vi "参数设置页.vi"() -> ()   [LabVIEW 2016, in "斯坦道总磷.lvlib"]
uses:
  <vilib>/Plasmionique/MB Master/MB_Master/MB_Master.lvclass
  <vilib>/ptbypt/NI_PtbyPt.lvlib
panel:
  in  "简易流程周期设置":cluster{"switch button":bool, "设置按钮":bool}
  out "连接状态":bool
  in  "标样核查自动补测":bool caption="通讯连接"
  in  "跨度核查自动补测":bool caption="通讯连接"
  in  "零点核查自动补测":bool caption="通讯连接"
  in  "标样核查标液偏差":dbl caption="标样核查标液偏差："
  in  "跨度核查标液偏差":dbl caption="跨度核查标液偏差："
  in  "零点核查标液偏差":dbl caption="零点核查标液偏差："
  out "低量程上限":dbl caption="低量程上限："
  in  "简易流程路径":path=path "data/流程.xml"
  out "数据刷新时间":string
  in  "通讯连接":bool=TRUE
  out "MB table":enum32{"Serial", "TCP"}(tab)
  in  "请选择串口:":refnum<visa-resource-name>
  in  "IP":string="127.0.0.1"
  in  "PORT":string="1001"
  in  "通信方式选择":enum16{"串口", "TCP"}(ring)
  in  "盐度自动补偿：":bool
  out "盐度补偿值":dbl caption="盐度补偿值："
  in  "刷新":bool
  in  "测量模式":T1(ring)
  in  "参数下拉列表":u16(ring)
  in  "量程下拉列表":enum16{"低量程", "高量程"}(ring)
  in  "测试流程路径":path=path "data/流程.xml"
  in  "标样核查量程模式":T2 caption="标样核查："
  in  "加标回收量程模式":T2 caption="加标回收："
  in  "跨度核查量程模式":T2 caption="跨度核查："
  in  "零点核查量程模式":T2 caption="零点核查："
  in  "水样测试量程模式":T2 caption="水样测试："
  out "稀释度":dbl caption="稀释度："
  out "阈值（高->低）":dbl caption="阈值（高->低）："
  out "阈值（低->高）":dbl caption="阈值（低->高）："
  out "量程下限":dbl caption="量程下限："
  out "高量程上限":dbl caption="高量程上限："
  out "检出限":dbl caption="检出限："
  out "曲线截距":dbl caption="曲线截距：" format="%#.6f"
  out "曲线斜率":dbl caption="曲线斜率：" format="%#.6f"
  out "二次多项式系数":dbl caption="二次多项式系数：" format="%#.6f"
  out "消解时长":dbl caption="消解时长："
  out "消解温度":dbl caption="消解温度："
  out "测量精度":u16 caption="测量精度："
  in  "标样核查标液浓度":dbl caption="标样核查标液浓度："
  in  "跨度核查标液浓度":dbl caption="跨度核查标液浓度："
  in  "零点核查标液浓度":dbl caption="零点核查标液浓度："
  in  "跨度值":dbl caption="跨度值："
  # "日质控设置"
  # "关键参数"
  # "连接设置"
  # "mg/L"
  # "mg/L"
  # "mg/L"
  # "mg/L"
  # "±"
  # "%"
  # "%"
  # "流程设置"
  # "简易流程周期设置"
  # "自动测试量程设置"
  # "设置："
  # "mg/L"
  # "ppt"
  # "mg/L"
  # "mg/L"
  # "mg/L"
  # "mg/L"
  # "mg/L"
  # "min"
  # "℃"
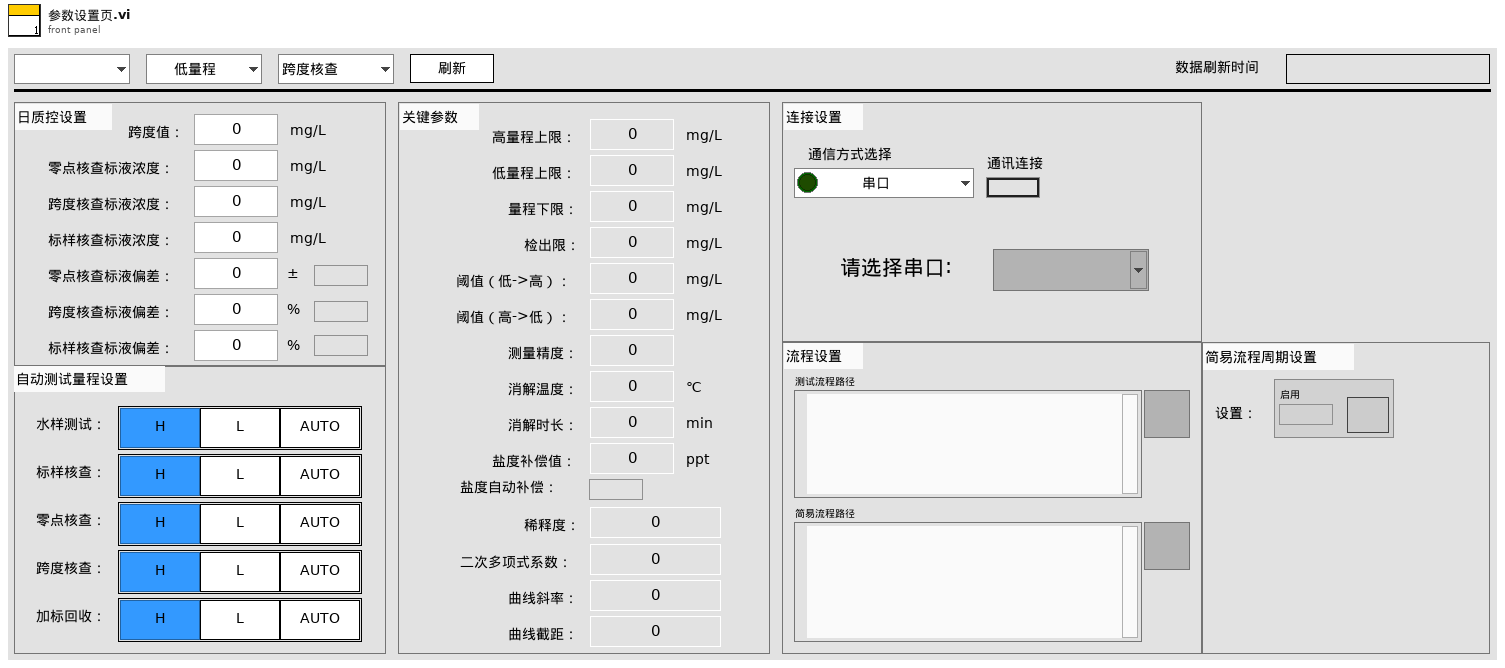
[diagram p1: front panel]
types:
  T1 = enum16{"跨度核查", "水样测量", "零点核查", "标样核查", "加标回收", "快捷测试", "空白校准", "标样校准"}
  T2 = typedef "斯坦道总磷.lvlib/量程模式.ctl" = enum32{"H", "L", "AUTO"}
  T3 = typedef "Cleaning cycle.lvclass/周期项.ctl" = cluster{"时":i32, "分":i32, "频次":string, "id":i32, "参数":string, "simpleflowid":i32, "简易流程名称":string}
  T4 = cluster{"系统时间":timestamp, "工作状态":u16, "测量模式":enum16{"待机", "连续模式", "周期模式", "定点模式", "受控模式", "手动模式"}, "告警代码":u16, "故障代码":u16, "日志代码":u16, "软件版本":u16, "F0":sgl, "F1":sgl, "F2":sgl, "F3":sgl, "T":sgl, "H":sgl, "id":u16, "flowid":u16, "量程":u16, "总磷控温温度1":sgl, "营养盐控温温度2":sgl, "ADC":sgl, "结果值":sgl, "运行时间":u16, "步骤详情":string, "步骤流程":string}
  T5 = typedef "LVStringsAndValuesArrayTypeDef_U16.ctl" = cluster{"String":string, "Value":u16}[]
  T6 = enum8{"Enabled", "Disabled", "Disabled and Grayed Out"}
  T7 = cluster{"测量精度":u16, "检出限":dbl, "上限":dbl, "下限":dbl, "阈值（低->高）":dbl, "阈值（高->低）":dbl, "稀释度":dbl}
  T8 = typedef "操作日志字段定义.ctl" = cluster{"时间":timestamp, "参数":string, "日志信息":string, "流程参数":string}
  T9 = typedef "SingleStepTestV3.lvlib/SingleStepTestV3.lvclass/仪器版本.ctl" = enum16{"V3.1版", "V4版", "V3版", "V4.2版"}
  T10 = typedef "斯坦道总磷.lvlib/V3.1版外设参数.ctl" = cluster{"泵类型":u8, "进样速度":u32, "出样速度":u32, "泵阀量":u8, "阀方向":u8, "光谱仪类型":u8, "光谱采样次数":u8, "氙灯次数":u8, "B":u16, "C":u16, "D":u16, "E":u16, "B_COD":u16, "C_COD":u16, "D_COD":u16, "E_COD":u16, "G":u16, "M":u16, "N":u16, "氨氮注射泵控温下限":sgl, "氨氮注射泵控温上限":sgl, "总氮注射泵控温下限":sgl, "总氮注射泵控温上限":sgl, "消解温度下限":sgl, "消解温度上限":sgl, "加热10s限值":sgl, "KP":sgl, "KI":sgl, "KD":sgl, "高温高压阀开阀温度":sgl, "总氮x公式0":u8, "总氮x公式1":sgl, "总氮x公式2":sgl, "总磷浊度稀释系数":sgl, "总磷浊度补偿权重1":sgl, "总磷浊度补偿权重2":sgl, "盐度系数":sgl, "氨氮补偿系数1":sgl, "氨氮补偿系数2":sgl}
  T11 = typedef "斯坦道总磷.lvlib/V4版外设参数.ctl" = cluster{"泵类型":u8, "注射泵正常速度":u32, "注射泵慢速":u32, "阀型号":u8, "res":u8, "光谱仪类型":u8, "光谱采样次数":u8, "氙灯次数":u8, "B":u16, "C":u16, "D":u16, "E":u16, "B_COD":u16, "C_COD":u16, "D_COD":u16, "E_COD":u16, "G":u16, "M":u16, "N":u16, "降温下限":sgl, "降温上限":sgl, "恒温温度下限":sgl, "恒温温度上限":sgl, "消解温度下限":sgl, "消解温度上限":sgl, "加热10s限值":sgl, "KP":sgl, "KI":sgl, "KD":sgl, "高温高压阀开阀温度":sgl, "总氮x公式0":u8, "总氮x公式1":sgl, "总氮x公式2":sgl, "总磷浊度稀释系数":sgl, "总磷浊度补偿权重1":sgl, "总磷浊度补偿权重2":sgl, "盐度系数":sgl, "氨氮补偿系数1":sgl, "氨氮补偿系数2":sgl, "缺试剂传感器阈值":u16}
  T12 = typedef "斯坦道总磷.lvlib/V4.2版外设参数.ctl" = cluster{"工作模式":u16, "泵类型":u16, "阀型号":u16, "注射泵进样速度":u16, "注射泵出样速度":u16, "注射泵滴定速度":u16, "res":u16, "注射泵慢速":u16, "光谱仪类型":u16, "光谱采样次数":u16, "氙灯次数":u16, "B":u16, "C":u16, "D":u16, "E":u16, "B_COD":u16, "C_COD":u16, "D_COD":u16, "E_COD":u16, "G":u16, "M":u16, "N":u16, "温度校准参数":sgl, "降温温度":sgl, "恒温温度":sgl, "消解温度":sgl, "高温高压阀开阀温度":sgl, "加热超时时间":sgl, "KP":sgl, "KI":sgl, "KD":sgl, "消解PID积分上限":sgl, "恒温PID积分上限":sgl, "PID积分下限":sgl, "缺试剂传感器阈值":u16, "滴定延时":u16, "滴定斜率阈值":sgl, "总氮x公式0":u16, "总氮x公式1":sgl, "总氮x公式2":sgl, "总磷浊度稀释系数":sgl, "总磷浊度补偿权重1":sgl, "总磷浊度补偿权重2":sgl, "盐度系数":sgl, "氨氮补偿系数1":sgl, "氨氮补偿系数2":sgl}
  T13 = typedef "斯坦道总磷.lvlib/V3版外设参数.ctl" = cluster{"泵类型":u8, "进样速度":u32, "出样速度":u32, "泵阀量":u8, "光谱仪类型":u8, "光谱采样次数":u8, "氙灯次数":u8, "B":u16, "C":u16, "D":u16, "E":u16, "B_COD":u16, "C_COD":u16, "D_COD":u16, "E_COD":u16, "G":u16, "M":u16, "N":u16, "氨氮注射泵控温下限":sgl, "氨氮注射泵控温上限":sgl, "总氮注射泵控温下限":sgl, "总氮注射泵控温上限":sgl, "消解温度下限":sgl, "消解温度上限":sgl, "加热10s限值":sgl, "高温高压阀开阀温度":sgl, "总氮x公式0":u8, "总氮x公式1":sgl, "总氮x公式2":sgl, "总磷浊度稀释系数":sgl, "总磷浊度补偿权重1":sgl, "总磷浊度补偿权重2":sgl, "盐度系数":sgl, "氨氮补偿系数1":sgl, "氨氮补偿系数2":sgl}
  T14 = cluster{"水样测试量程模式":T2, "零点核查量程模式":T2, "跨度核查量程模式":T2, "加标回收量程模式":T2, "标样核查量程模式":T2}
  T15 = cluster{"总磷":dbl, "总氮":dbl, "氨氮":dbl, "磷酸盐":dbl, "硝氮":dbl, "亚硝氮":dbl, "硅酸盐":dbl, "硫化物":dbl, "COD":dbl, "氟化物":dbl, "CODMn":dbl}
  T16 = cluster{"总磷跨度值":dbl, "总磷零点标准液浓度":dbl, "总磷跨度标准液浓度":dbl, "总磷标准液标准浓度":dbl, "总氮跨度值":dbl, "总氮零点标准液浓度":dbl, "总氮跨度标准液浓度":dbl, "总氮标准液标准浓度":dbl, "COD跨度值":dbl, "COD零点标准液浓度":dbl, "COD跨度标准液浓度":dbl, "COD标准液标准浓度":dbl, "氨氮跨度值":dbl, "氨氮零点标准液浓度":dbl, "氨氮跨度标准液浓度":dbl, "氨氮标准液标准浓度":dbl, "磷酸盐跨度值":dbl, "磷酸盐零点标准液浓度":dbl, "磷酸盐跨度标准液浓度":dbl, "磷酸盐标准液标准浓度":dbl, "硝氮跨度值":dbl, "硝氮零点标准液浓度":dbl, "硝氮跨度标准液浓度":dbl, "硝氮标准液标准浓度":dbl, "亚硝氮跨度值":dbl, "亚硝氮零点标准液浓度":dbl, "亚硝氮跨度标准液浓度":dbl, "亚硝氮标准液标准浓度":dbl, "硫化物跨度值":dbl, "硫化物零点标准液浓度":dbl, "硫化物跨度标准液浓度":dbl, "硫化物标准液标准浓度":dbl, "硅酸盐跨度值":dbl, "硅酸盐零点标准液浓度":dbl, "硅酸盐跨度标准液浓度":dbl, "硅酸盐标准液标准浓度":dbl, "总磷零点标准液偏差":dbl, "总磷跨度标准液偏差":dbl, "总磷标准液标准偏差":dbl, "总氮零点标准液偏差":dbl, "总氮跨度标准液偏差":dbl, "总氮标准液标准偏差":dbl, "COD零点标准液偏差":dbl, "COD跨度标准液偏差":dbl, "COD标准液标准偏差":dbl, "氨氮零点标准液偏差":dbl, "氨氮跨度标准液偏差":dbl, "氨氮标准液标准偏差":dbl, "磷酸盐零点标准液偏差":dbl, "磷酸盐跨度标准液偏差":dbl, "磷酸盐标准液标准偏差":dbl, "硝氮零点标准液偏差":dbl, "硝氮跨度标准液偏差":dbl, "硝氮标准液标准偏差":dbl, "亚硝氮零点标准液偏差":dbl, "亚硝氮跨度标准液偏差":dbl, "亚硝氮标准液标准偏差":dbl, "硫化物零点标准液偏差":dbl, "硫化物跨度标准液偏差":dbl, "硫化物标准液标准偏差":dbl, "硅酸盐零点标准液偏差":dbl, "硅酸盐跨度标准液偏差":dbl, "硅酸盐标准液标准偏差":dbl, "氟化物跨度值":dbl, "氟化物零点标准液浓度":dbl, "氟化物跨度标准液浓度":dbl, "氟化物标准液标准浓度":dbl, "氟化物零点标准液偏差":dbl, "氟化物跨度标准液偏差":dbl, "氟化物标准液标准偏差":dbl, "CODMn跨度值":dbl, "CODMn零点标准液浓度":dbl, "CODMn跨度标准液浓度":dbl, "CODMn标准液标准浓度":dbl, "CODMn零点标准液偏差":dbl, "CODMn跨度标准液偏差":dbl, "CODMn标准液标准偏差":dbl}
  T17 = cluster{"水样测试量程模式":enum16{"H", "L", "AUTO"}, "空白核查量程模式":enum16{"H", "L", "AUTO"}, "跨度核查量程模式":enum16{"H", "L", "AUTO"}, "加标回收量程模式":enum16{"H", "L", "AUTO"}, "标样核查量程模式":enum16{"H", "L", "AUTO"}}
  T18 = cluster{"水样测试量程模式":u16, "空白核查量程模式":u16, "跨度核查量程模式":u16, "加标回收量程模式":u16, "标样核查量程模式":u16}
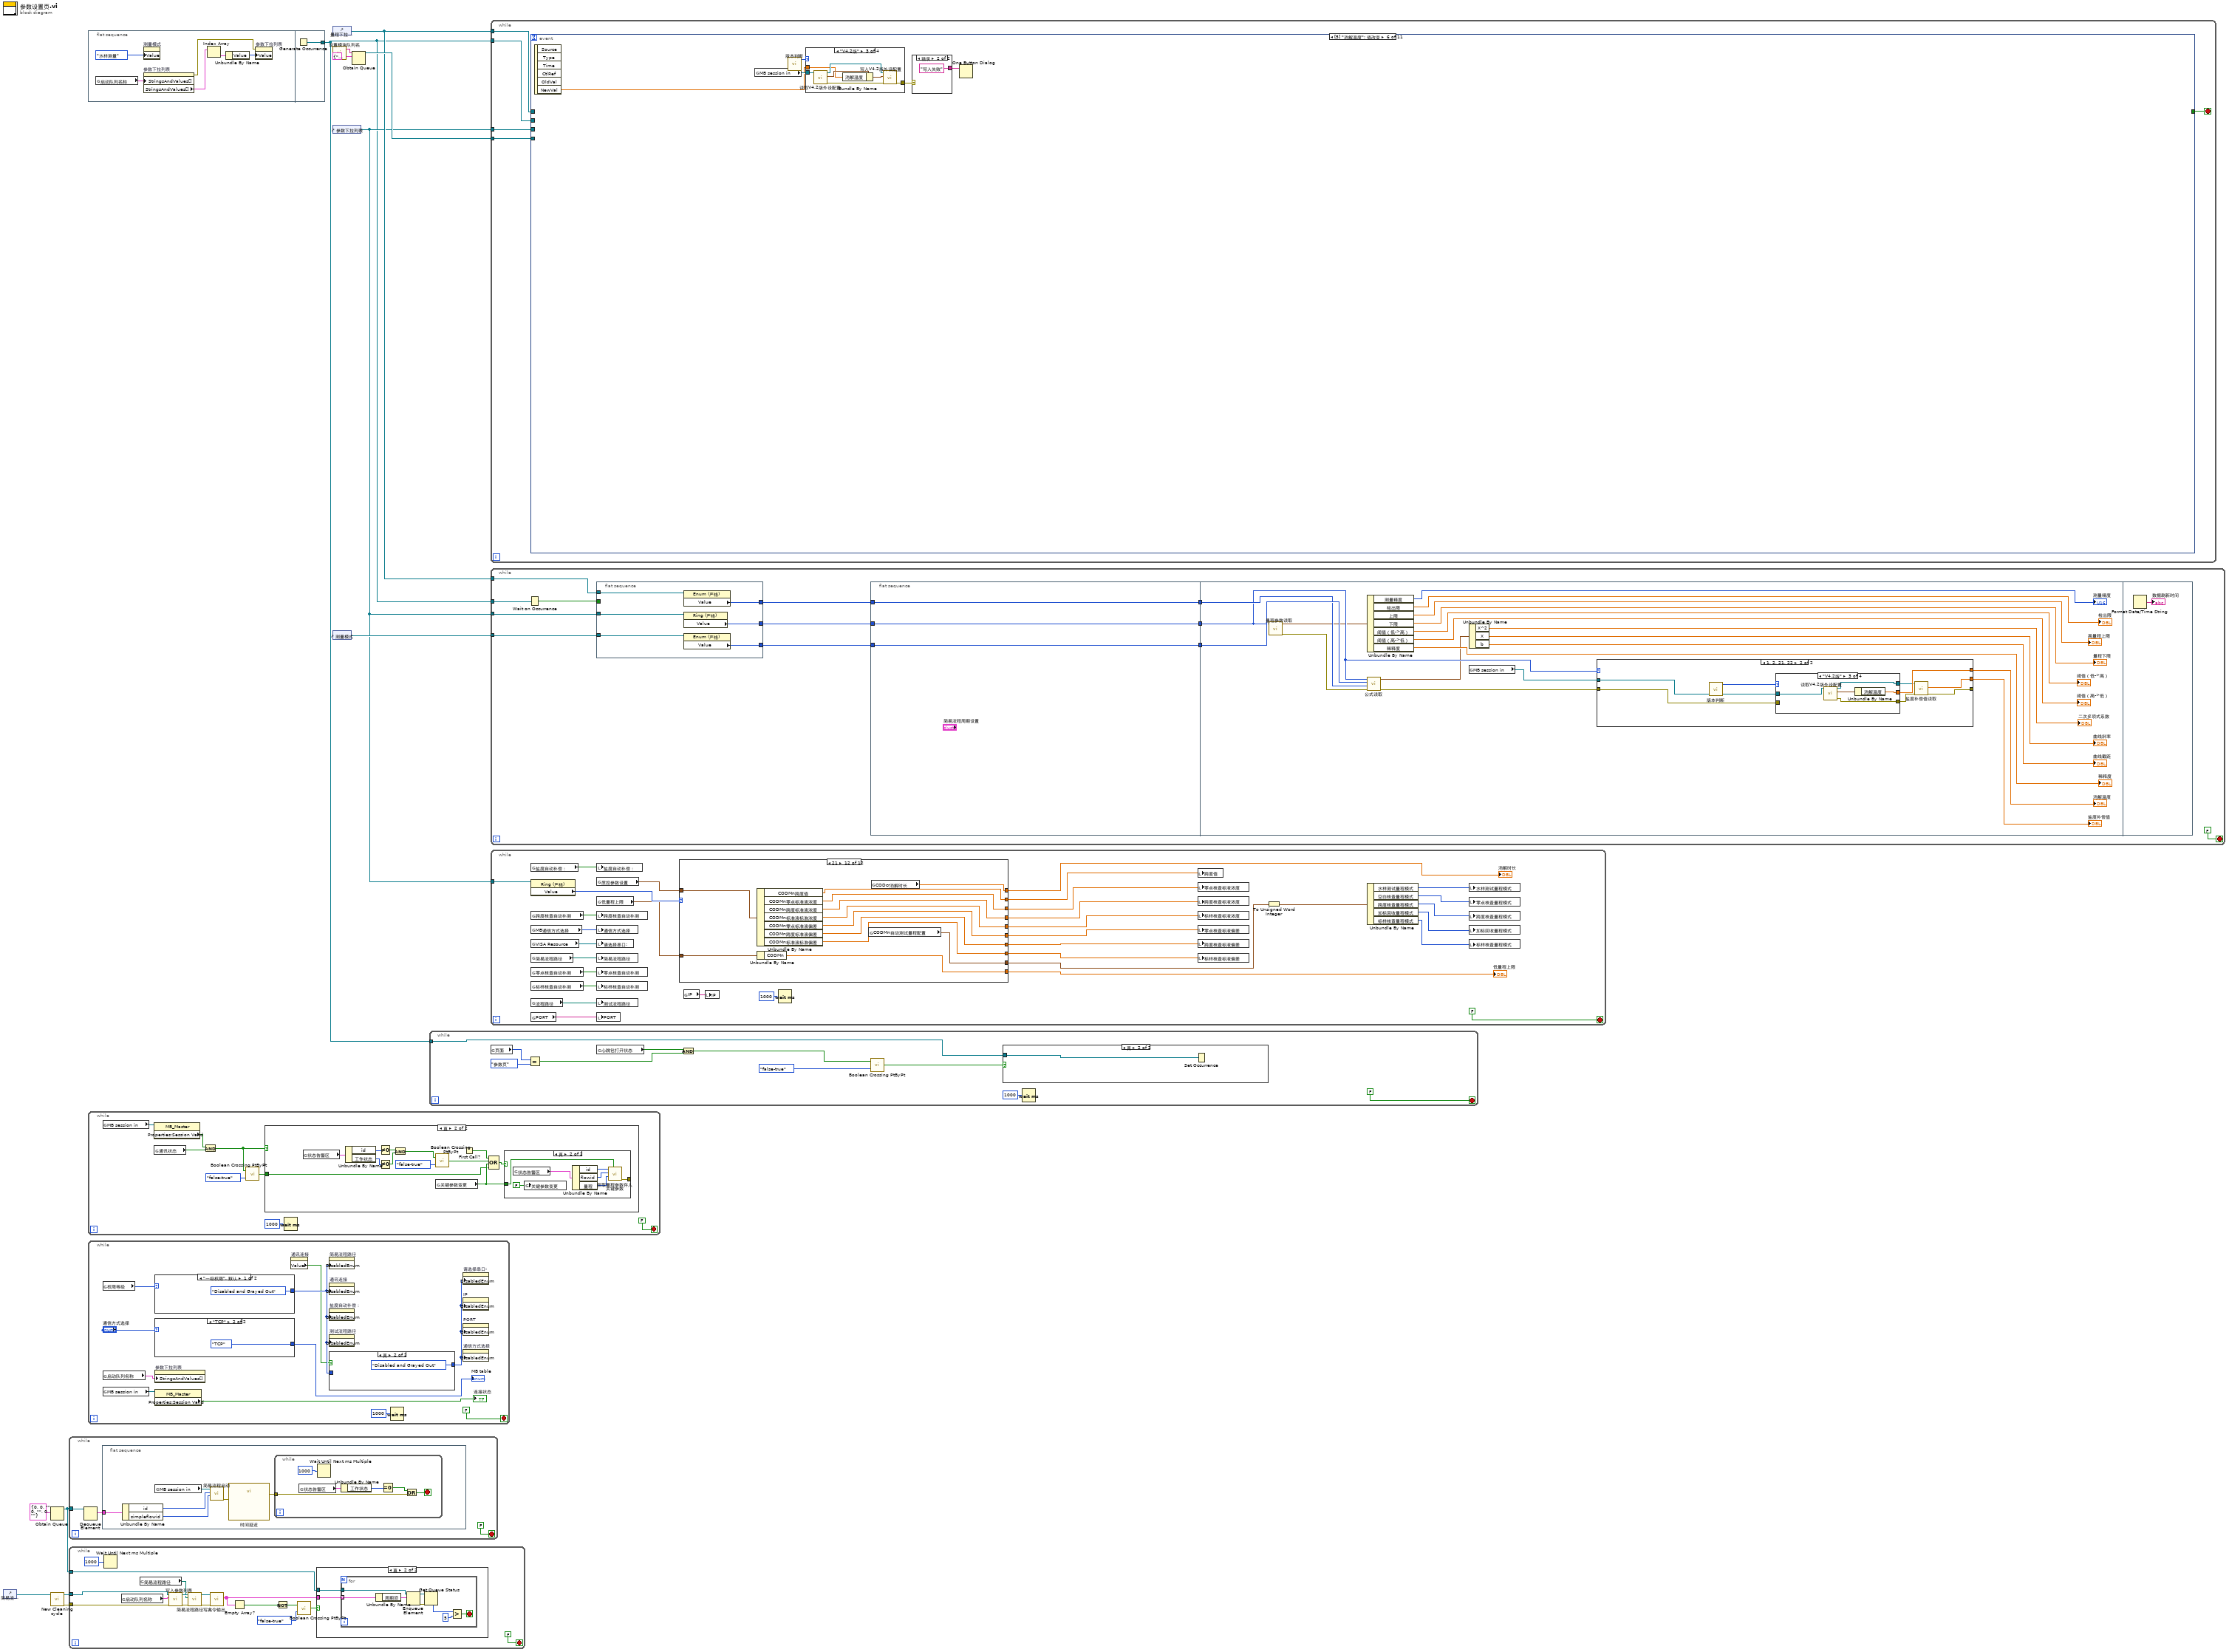
[diagram p0: block diagram]
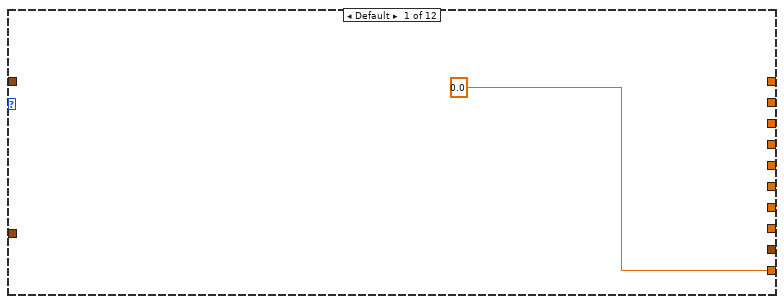
[diagram p6: hidden frame]
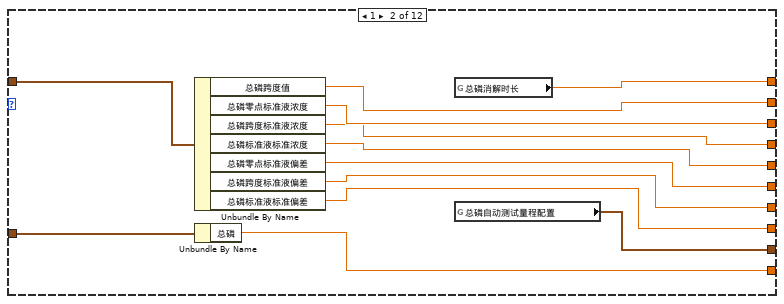
[diagram p7: hidden frame]
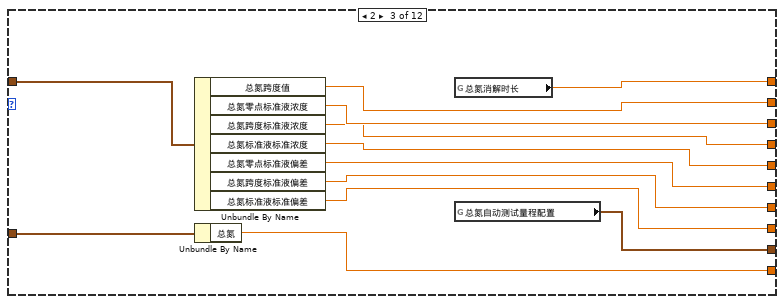
[diagram p8: hidden frame]
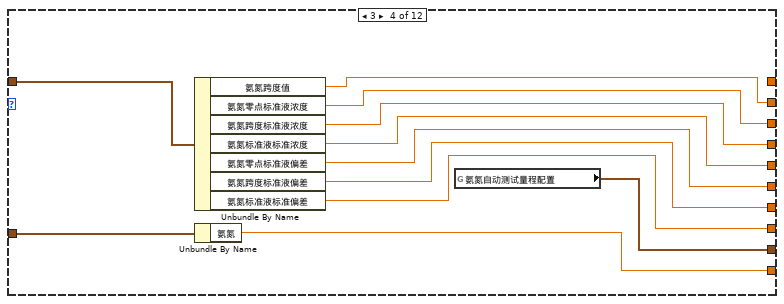
[diagram p9: hidden frame]
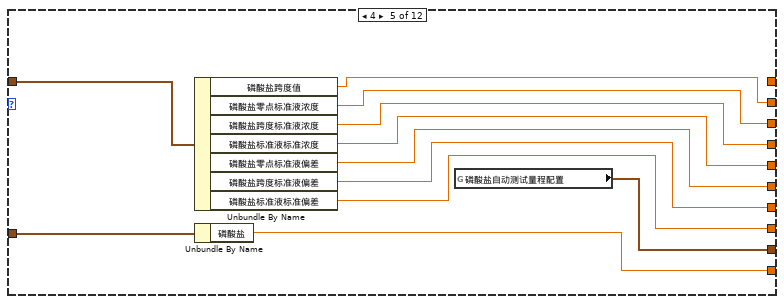
[diagram p10: hidden frame]
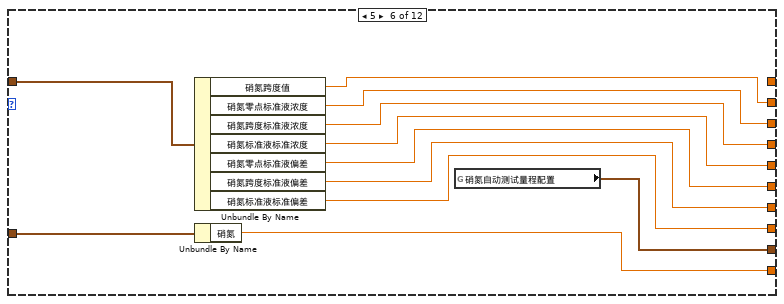
[diagram p11: hidden frame]
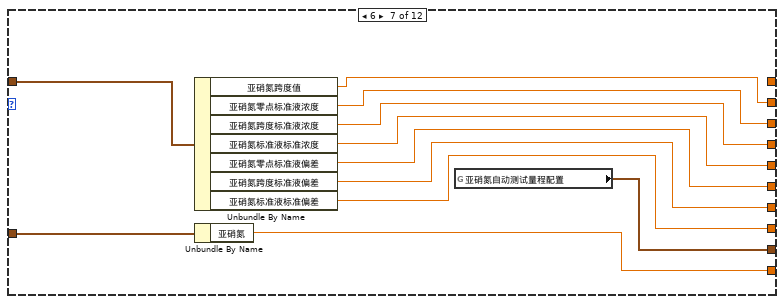
[diagram p12: hidden frame]
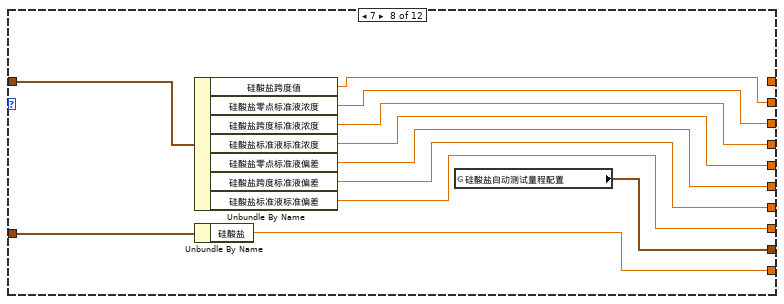
[diagram p13: hidden frame]
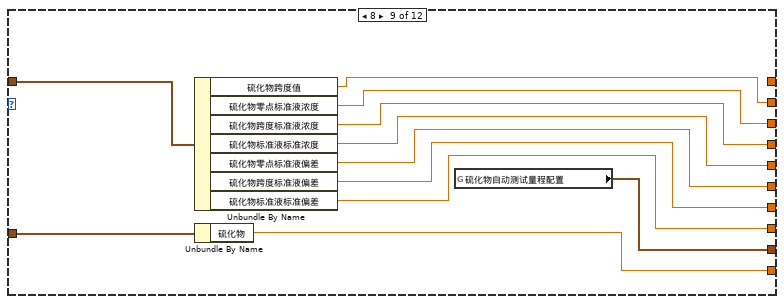
[diagram p14: hidden frame]
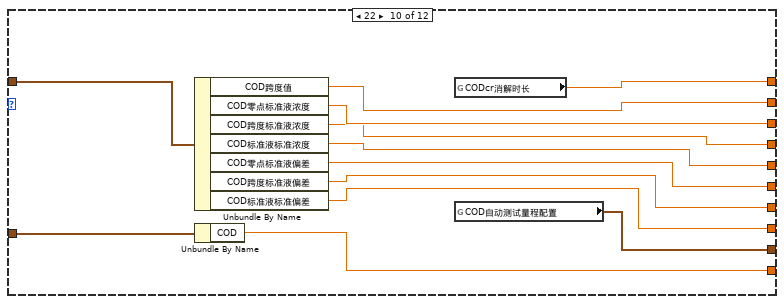
[diagram p15: hidden frame]
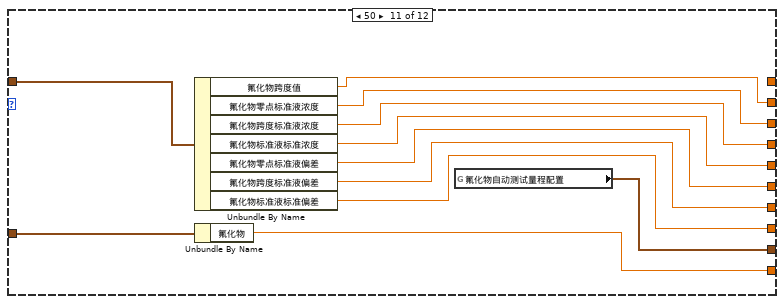
[diagram p16: hidden frame]
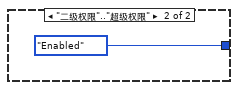
[diagram p17: hidden frame]
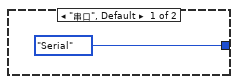
[diagram p18: hidden frame]
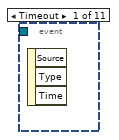
[diagram p20: hidden frame]
diagram:
  n1 = control-ref of="简易流程周期设置"() -> (w3:refnum<vi>)
  n2 = Obtain Queue(element data type=T3 {"时"=0, "分"=0, "频次"="", "id"=0, "参数"="", "simpleflowid"=0, "简易流程名称"=""} ("周期项")) -> (queue out=w1:refnum<queue>)  [unwired: 4 in, 2 out]
  n3 = call "New Cleaning cycle.vi"("Reference"=w3) -> ("error out"=w4:errorcluster, "Cleaningcycle out"=w5:refnum<class "Cleaning cycle.lvclass">)  [unwired: 9 in]
  n4 = while {
    tunnel: w1 -> [w15]
    stop <- FALSE stop-if-true
    n5 = Dequeue Element(queue=w15) -> (element=w14:T3)  [unwired: 2 in, 3 out]
    n6 = flat-sequence {
      tunnel: w14 -> [w20]
      frame #0 {
        n7 = Unbundle By Name(w20) -> ("id"=w18:i32, "simpleflowid"=w19:i32)
        n8 = global read "VAR总磷总氮全局变量.vi" "MB session in"() -> (w21:refnum<class "MB_Master.lvclass">)
        n9 = call "简易流程启动.vi"("简易流程"=w19, "参数Id"=w18, "MB session in"=w21) -> ("error out"=w17:errorcluster)  [unwired: 7 in, 1 out]
        n10 = call "时间延迟"("error in (no error)"=w17) -> ("error out"=w16:errorcluster)  [unwired: 10 in]
        n11 = while {
          tunnel: w16 -> [w23]
          stop <- w22 stop-if-true
          n12 = global read "VAR总磷总氮全局变量.vi" "状态告警区"() -> (w26:T4)
          n13 = Wait Until Next ms Multiple(millisecond multiple=u32 1000 ("毫秒倍数")) -> ()  [unwired: 1 out]
          n14 = Unbundle By Name(w26) -> ("工作状态"=w25:u16)
          n15 = Equal To 0?(x=w25) -> (x = 0?=w24:bool)
          n16 = Or(x=w24, y=w23) -> (x .or. y?=w22:bool)
        }
      }
    }
  }
  n17 = while {
    tunnel: w5 -> [w43]
    tunnel: w4 -> [w42]
    tunnel: w1 -> [w29]
    stop <- FALSE stop-if-true
    n18 = Wait Until Next ms Multiple(millisecond multiple=u32 1000 ("毫秒倍数")) -> ()  [unwired: 1 out]
    n19 = global read "model config var.vi" "启动队列名称"() -> (w39:cluster{"String":string, "Value":u16}[])
    n20 = global read "总磷总氮断电保存全局变量.vi" "简易流程路径"() -> (w38:path)
    n21 = call "写入参数列表.vi"("error in (no error)"=w42, "参数列表"=w39, "Cleaningcycle 输入"=w43) -> ("error out"=w41:errorcluster, "Cleaningcycle 输出"=w40:refnum<class "Cleaning cycle.lvclass">)  [unwired: 7 in]
    n22 = call "简易流程路径写入.vi"("error in (no error)"=w41, "简易流程路径"=w38, "Cleaningcycle 输入"=w40) -> ("error out"=w36:errorcluster, "Cleaningcycle 输出"=w37:refnum<class "Cleaning cycle.lvclass">)  [unwired: 7 in]
    n23 = call "命令输出.vi"("error in (no error)"=w36, "Cleaningcycle 输入"=w37) -> ("命令"=w31:cluster{"触发":bool, "周期项":T3}[])  [unwired: 7 in, 2 out]
    n24 = Empty Array?(array=w31) -> (empty?=w35:bool)
    n25 = Not(x=w35) -> (.not. x?=w34:bool)
    n26 = call <vilib>:"Boolean Crossing PtByPt.vi"("direction"=enum16{"either", "false-true", "true-false"}."false-true", "input"=w34) -> ("crossing"=w32:bool)  [unwired: 1 in]
    n27 = case shown="真" w32 {
      tunnel: w31 -> [_ w45]
      tunnel: w29 -> [_ w44]
      frame False {
      }
      frame True {
        n28 = for {
          tunnel: w45 -> [w53] mode=indexing
          tunnel: w44 -> [w51]
          stop <- w46 stop-if-true
          n29 = Unbundle By Name(w53) -> ("周期项"=w52:T3)
          n30 = Enqueue Element(queue=w51, element=w52) -> (queue out=w50:refnum<queue>, error out=w49:errorcluster)  [unwired: 2 in, 1 out]
          n31 = Get Queue Status(queue=w50, error in (no error)=w49) -> (# elements in queue=w48:i32)  [unwired: 1 in, 7 out]
          n32 = Greater?(x=w48, y=5) -> (0:w46:bool)
        }
      }
    }
  }
  n33 = flat-sequence {
    tunnel: [w60] -> w6
    frame #0 {
      n34 = global read "model config var.vi" "启动队列名称"() -> (w55:cluster{"String":string, "Value":u16}[])
      n35 = property on="测量模式" class="Enum (严格)"("Value"=T1."水样测量" ("测量模式")) -> ()  [unwired: 2 in, 2 out]
      n36 = property on="参数下拉列表" class="Ring (严格)"("StringsAndValues[]"=w55) -> (error out=w58:errorcluster, "StringsAndValues[]"=w56:T5)  [unwired: 2 in, 1 out]
      n37 = Index Array(array=w56) -> (element=w57:cluster{"String":string, "Value":u16})  [unwired: 1 in]
      n38 = Unbundle By Name(w57) -> ("Value"=w59:u16)
      n39 = property on="参数下拉列表" class="Ring (严格)"(error in=w58, "Value"=w59) -> ()  [unwired: 1 in, 2 out]
    }
    frame #1 {
      n40 = Generate Occurrence() -> (w60:refnum<k4>)
    }
  }
  n41 = while {
    stop <- FALSE stop-if-true
    n42 = global read "VAR总磷总氮全局变量.vi" "MB session in"() -> (w65:refnum<class "MB_Master.lvclass">)
    n43 = property class="MB_Master"(reference=w65) -> ("Properties:Session Valid"=w64:bool)  [unwired: 1 in, 2 out]
    n44 = global read "VAR总磷总氮全局变量.vi" "通讯状态"() -> (w67:bool)
    n45 = And(x=w64, y=w67) -> (x .and. y?=w62:bool)
    n46 = call <vilib>:"Boolean Crossing PtByPt.vi"("direction"=enum16{"either", "false-true", "true-false"}."false-true", "input"=w62) -> ("crossing"=w61:bool)  [unwired: 1 in]
    n47 = case shown="真" w62 {
      tunnel: w61 -> [_ w70]
      frame False {
      }
      frame True {
        n48 = global read "VAR总磷总氮全局变量.vi" "状态告警区"() -> (w80:T4)
        n49 = Unbundle By Name(w80) -> ("id"=w74:u16, "工作状态"=w79:u16)
        n50 = Not Equal To 0?(x=w74) -> (x != 0?=w75:bool)
        n51 = Not Equal To 0?(x=w79) -> (x != 0?=w76:bool)
        n52 = And(x=w75, y=w76) -> (x .and. y?=w77:bool)
        n53 = call <vilib>:"Boolean Crossing PtByPt.vi"("direction"=enum16{"either", "false-true", "true-false"}."false-true", "input"=w77) -> ("crossing"=w73:bool)  [unwired: 1 in]
        n54 = global read "VAR总磷总氮全局变量.vi" "关键参数变更"() -> (w71:bool)
        n55 = First Call?() -> (First Call?: T/F=w69:bool)
        n56 = Compound Arithmetic op=OR ("复合运算")(w69, w73, w71, w70) -> (w72:bool)
        n57 = case shown="真" w72 {
          tunnel: [_ w87] -> _
          tunnel: w71 -> [_ w82]
          frame False {
          }
          frame True {
            n58 = global read "VAR总磷总氮全局变量.vi" "状态告警区"() -> (w86:T4)
            n59 = global write "VAR总磷总氮全局变量.vi" "关键参数变更"(FALSE ("关键参数变更")) -> ()
            n60 = Unbundle By Name(w86) -> ("id"=w85:u16, "flowid"=w84:u16, "量程"=w83:u16)
            n61 = call "获取量程参数存入关键参数.vi"("关键参数变更"=w82, "量程"=w83, "flowid"=w84, "id"=w85) -> ("error out"=w87:errorcluster)  [unwired: 7 in]
          }
        }
      }
    }
    n62 = Wait (ms)(milliseconds to wait=u32 1000 ("等待时间（毫秒）")) -> ()  [unwired: 1 out]
  }
  n63 = while {
    stop <- FALSE stop-if-true
    n64 = global read "VAR总磷总氮全局变量.vi" "权限等级"() -> (w92:enum16{"一级权限", "二级权限", "三级权限", "超级权限"})
    n65 = global read "model config var.vi" "启动队列名称"() -> (w90:cluster{"String":string, "Value":u16}[])
    n66 = global read "VAR总磷总氮全局变量.vi" "MB session in"() -> (w97:refnum<class "MB_Master.lvclass">)
    n67 = case shown="\"一级权限\", 默认" w92 {
      tunnel: [T6."Disabled and Grayed Out" ("禁用") T6."Enabled" ("禁用")] -> w91
      frame "一级权限", Default {
      }
      frame "二级权限".."超级权限" {
      }
    }
    n68 = case shown="\"TCP\"" "通信方式选择" {
      tunnel: [enum32{"Serial", "TCP"}."Serial" ("MB table") enum32{"Serial", "TCP"}."TCP" ("MB table")] -> w94
      frame "串口", Default {
      }
      frame "TCP" {
      }
    }
    "MB table" <- w94
    n69 = property on="参数下拉列表" class="Ring (严格)"("StringsAndValues[]"=w90) -> ()  [unwired: 2 in, 2 out]
    n70 = property class="MB_Master"(reference=w97) -> ("Properties:Session Valid"=→"连接状态":bool)  [unwired: 1 in, 2 out]
    n71 = property on="通讯连接" class="Bool (严格)"() -> ("Value"=w88:bool)  [unwired: 2 in, 2 out]
    n72 = property on="简易流程路径" class="Path"("DisabledEnum"=w91) -> ()  [unwired: 2 in, 2 out]
    n73 = property on="通讯连接" class="Bool (严格)"("DisabledEnum"=w91) -> ()  [unwired: 2 in, 2 out]
    n74 = property on="盐度自动补偿：" class="Bool (严格)"("DisabledEnum"=w91) -> ()  [unwired: 2 in, 2 out]
    n75 = property on="测试流程路径" class="Path"("DisabledEnum"=w91) -> ()  [unwired: 2 in, 2 out]
    n76 = case shown="真" w88 {
      tunnel: [w103 T6."Disabled and Grayed Out" ("禁用")] -> w95
      tunnel: w91 -> [w103 _]
      frame False {
      }
      frame True {
      }
    }
    n77 = Wait (ms)(milliseconds to wait=u32 1000 ("等待时间（毫秒）")) -> ()  [unwired: 1 out]
    n78 = property on="请选择串口:" class="VISAName"("DisabledEnum"=w95) -> ()  [unwired: 2 in, 2 out]
    n79 = property on="IP" class="Str"("DisabledEnum"=w95) -> ()  [unwired: 2 in, 2 out]
    n80 = property on="PORT" class="Str"("DisabledEnum"=w95) -> ()  [unwired: 2 in, 2 out]
    n81 = property on="通信方式选择" class="Enum (严格)"("DisabledEnum"=w95) -> ()  [unwired: 2 in, 2 out]
  }
  n82 = control-ref of="量程下拉列表"() -> (w8:refnum<vi>)
  n83 = call "设置模块队列名.vi"() -> ("Msg"=w11:string)  [unwired: 5 in]
  n84 = control-ref of="参数下拉列表"() -> (w7:refnum<vi>)
  n85 = control-ref of="测量模式"() -> (w9:refnum<vi>)
  n86 = Obtain Queue(name (unnamed)=w11, element data type=cluster{"命令":string, "data":variant} {"命令"="", "data"=variant}) -> (queue out=w10:refnum<queue>)  [unwired: 3 in, 2 out]
  n87 = while {
    tunnel: w6 -> [w111]
    stop <- FALSE stop-if-true
    n88 = global read "VAR总磷总氮全局变量.vi" "页面"() -> (w113:enum16{"主页", "参数页", "校准页"})
    n89 = Equal?(x=w113, y=enum16{"主页", "参数页", "校准页"}."参数页" ("页面")) -> (x = y?=w112:bool)
    n90 = global read "VAR总磷总氮全局变量.vi" "心跳包打开状态"() -> (w107:bool)
    n91 = And(x=w107, y=w112) -> (x .and. y?=w108:bool)
    n92 = call <vilib>:"Boolean Crossing PtByPt.vi"("direction"=enum16{"either", "false-true", "true-false"}."false-true", "input"=w108) -> ("crossing"=w106:bool)  [unwired: 1 in]
    n93 = case shown="真" w106 {
      tunnel: w111 -> [_ w115]
      frame False {
      }
      frame True {
        n94 = Set Occurrence(w115) -> ()
      }
    }
    n95 = Wait (ms)(milliseconds to wait=u32 1000 ("等待时间（毫秒）")) -> ()  [unwired: 1 out]
  }
  n96 = while {
    tunnel: w6 -> [w119]
    tunnel: w7 -> [w118]
    tunnel: w10 -> [w117]
    tunnel: w8 -> [w116]
    stop <- w120 stop-if-true
    n97 = event shown="[5] \"消解温度\": 值改变" {
      selector: _ -> [_ _ _ _ _ _ _ _ _ _ _]
      dyn-events: _ -> [_ _ _ _ _ _ _ _ _ _ _]
      timeout: _ -> [_ _ _ _ _ _ _ _ _ _ _]
      tunnel: [_ TRUE _ _ _ _ _ _ _ _ _] -> w120
      tunnel: w119 -> [_ _ w122 _ _ _ _ _ _ w201 _]
      tunnel: w118 -> [_ _ _ _ w141 _ _ _ _ w203 _]
      tunnel: w117 -> [_ _ _ _ _ _ _ _ _ _ w391]
      tunnel: w116 -> [_ _ _ _ _ _ _ _ _ _ _]
      event Timeout {
        n98 = event-data() -> ()  [unwired: 1 in, 3 out]
      }
      event Panel Close {
        n99 = event-data() -> ()  [unwired: 1 in, 4 out]
      }
      event "参数下拉列表", "量程下拉列表", "测量模式", "刷新": Value Change {
        n100 = event-data() -> ()  [unwired: 1 in, 6 out]
        n101 = Set Occurrence(w122) -> ()
      }
      event "跨度值", "零点核查标液浓度", "跨度核查标液浓度", "标样核查标液浓度", "消解温度", "消解时长", "检出限", "高量程上限", "量程下限", "阈值（低->高）", "阈值（高->低）", "稀释度", "低量程上限", "零点核查标液偏差", "跨度核查标液偏差", "标样核查标液偏差": Mouse Down {
        n102 = event-data() -> ("CtlRef"=w124:refnum<vi>)  [unwired: 1 in, 5 out]
        n103 = global read "VAR总磷总氮全局变量.vi" "权限等级"() -> (w123:enum16{"一级权限", "二级权限", "三级权限", "超级权限"})
        n104 = case shown="\"二级权限\"..\"超级权限\"" w123 {
          tunnel: w124 -> [_ w128]
          frame "一级权限", Default {
          }
          frame "二级权限".."超级权限" {
            n105 = property class="DigNum (严格)"(reference=w128) -> (reference out=w126:refnum<vi>, "Value"=w127:dbl)  [unwired: 1 in, 1 out]
            n106 = call "数字键盘.vi"("OldNumber"=w127) -> ("NewNumber"=w125:dbl)
            n107 = property class="DigNum (严格)"(reference=w126, "Val(Sgnl)"=w125) -> ()  [unwired: 1 in, 2 out]
          }
        }
      }
      event "测量精度", "检出限", "高量程上限", "量程下限", "阈值（低->高）", "阈值（高->低）", "稀释度": Value Change {
        n108 = event-data() -> ()  [unwired: 1 in, 6 out]
        n109 = local read "测量精度"() -> (w131:u16)
        n110 = local read "检出限"() -> (w135:dbl)
        n111 = local read "高量程上限"() -> (w137:dbl)
        n112 = local read "量程下限"() -> (w136:dbl)
        n113 = local read "阈值（低->高）"() -> (w134:dbl)
        n114 = local read "阈值（高->低）"() -> (w133:dbl)
        n115 = local read "稀释度"() -> (w132:dbl)
        n116 = property class="Ring (严格)"(reference=w141) -> ("Value"=w140:u16)  [unwired: 1 in, 2 out]
        n117 = Bundle By Name(cluster=T7 {"测量精度"=0, "检出限"=0.0, "上限"=0.0, "下限"=0.0, "阈值（低->高）"=0.0, "阈值（高->低）"=0.0, "稀释度"=0.0} ("量程参数写入"), "测量精度"=w131, "检出限"=w135, "上限"=w137, "下限"=w136, "阈值（低->高）"=w134, "阈值（高->低）"=w133, "稀释度"=w132) -> (w138:T7)
        n118 = call "量程参数写入.vi"("量程参数写入"=w138, "测量参数"=w140) -> ("error out"=w129:errorcluster)  [unwired: 8 in]
        n119 = case shown="无错误" w129 {
          tunnel: ["写入成功" "写入失败"] -> w130
          frame No Error {
            n120 = Get Date/Time In Seconds() -> (seconds since 1Jan1904=w144:timestamp)
            n121 = property on="参数下拉列表" class="Ring (严格)"() -> ("RingText.Text"=w142:string)  [unwired: 2 in, 2 out]
            n122 = Bundle By Name(cluster=T8 {"时间"=timestamp(0 s since 1904-01-01), "参数"="", "日志信息"="", "流程参数"=""} ("data in"), "时间"=w144, "参数"=w142, "日志信息"="关键参数变更") -> (w145:T8)
            n123 = call "总磷总氮操作日志.vi"("data in"=w145) -> ()  [unwired: 10 in, 1 out]
            n124 = global write "VAR总磷总氮全局变量.vi" "关键参数变更"(TRUE ("关键参数变更")) -> ()
          }
          frame Error {
          }
        }
        n125 = One Button Dialog(message=w130) -> ()  [unwired: 1 in, 1 out]
      }
      event "消解温度": Value Change {
        n126 = event-data() -> ("NewVal"=w151:dbl)  [unwired: 1 in, 5 out]
        n127 = global read "VAR总磷总氮全局变量.vi" "MB session in"() -> (w152:refnum<class "MB_Master.lvclass">)
        n128 = call "版本判断.vi"() -> ("仪器版本"=w153:T9)  [unwired: 11 in]
        n129 = case shown="\"V4.2版\"" w153 {
          tunnel: w152 -> [w161 w168 w175 w182]
          tunnel: w151 -> [w156 w164 w171 w178]
          tunnel: [w155 w162 w169 w176] -> w150
          frame "V3.1版", Default {
            n130 = call "读取V3.1外设配置.vi"("MB session in"=w161) -> ("error out"=w157:errorcluster, "外设配置"=w160:T10, "MB session out"=w159:refnum<class "MB_Master.lvclass">)  [unwired: 8 in]
            n131 = Bundle By Name(cluster=w160, "消解温度下限"=w156) -> (w158:T10)
            n132 = call "写入V3.1外设配置.vi"("error in (no error)"=w157, "外设配置"=w158, "MB session in"=w159) -> ("error out"=w155:errorcluster)  [unwired: 7 in, 1 out]
          }
          frame "V4版" {
            n133 = call "读取V4版外设配置.vi"("MB session in"=w168) -> ("error out"=w163:errorcluster, "外设配置"=w166:T11, "MB session out"=w167:refnum<class "MB_Master.lvclass">)  [unwired: 8 in]
            n134 = Bundle By Name(cluster=w166, "消解温度下限"=w164) -> (w165:T11)
            n135 = call "写入V4版外设配置.vi"("error in (no error)"=w163, "外设配置"=w165, "MB session in"=w167) -> ("error out"=w162:errorcluster)  [unwired: 7 in, 1 out]
          }
          frame "V4.2版" {
            n136 = call "读取V4.2版外设配置.vi"("MB session in"=w175) -> ("error out"=w170:errorcluster, "外设配置"=w173:T12, "MB session out"=w174:refnum<class "MB_Master.lvclass">)  [unwired: 8 in]
            n137 = Bundle By Name(cluster=w173, "消解温度"=w171) -> (w172:T12)
            n138 = call "写入V4.2版外设配置.vi"("error in (no error)"=w170, "外设配置"=w172, "MB session in"=w174) -> ("error out"=w169:errorcluster)  [unwired: 7 in, 1 out]
          }
          frame "V3版" {
            n139 = call "读取V3外设配置.vi"("MB session in"=w182) -> ("error out"=w177:errorcluster, "外设配置"=w180:T13, "MB session out"=w181:refnum<class "MB_Master.lvclass">)  [unwired: 8 in]
            n140 = Bundle By Name(cluster=w180, "消解温度下限"=w178) -> (w179:T13)
            n141 = call "写入V3外设配置.vi"("error in (no error)"=w177, "外设配置"=w179, "MB session in"=w181) -> ("error out"=w176:errorcluster)  [unwired: 7 in, 1 out]
          }
        }
        n142 = case shown="错误" w150 {
          tunnel: ["写入成功" "写入失败"] -> w154
          frame No Error {
          }
          frame Error {
          }
        }
        n143 = One Button Dialog(message=w154) -> ()  [unwired: 1 in, 1 out]
      }
      event "测量精度": Mouse Down {
        n144 = event-data() -> ("CtlRef"=w186:refnum<vi>)  [unwired: 1 in, 7 out]
        n145 = global read "VAR总磷总氮全局变量.vi" "权限等级"() -> (w185:enum16{"一级权限", "二级权限", "三级权限", "超级权限"})
        n146 = case shown="\"二级权限\"..\"超级权限\"" w185 {
          tunnel: w186 -> [_ w190]
          frame "一级权限", Default {
          }
          frame "二级权限".."超级权限" {
            n147 = property class="DigNum (严格)"(reference=w190) -> (reference out=w188:refnum<vi>, "Value"=w189:u16)  [unwired: 1 in, 1 out]
            n148 = call "数字键盘.vi"("OldNumber"=w189) -> ("NewNumber"=w187:dbl)
            n149 = property class="DigNum (严格)"(reference=w188, "Val(Sgnl)"=w187) -> ()  [unwired: 1 in, 2 out]
          }
        }
      }
      event "盐度补偿值": Mouse Down {
        n150 = event-data() -> ("CtlRef"=w192:refnum<vi>)  [unwired: 1 in, 3 out]
        n151 = global read "VAR总磷总氮全局变量.vi" "权限等级"() -> (w191:enum16{"一级权限", "二级权限", "三级权限", "超级权限"})
        n152 = case shown="\"二级权限\"..\"超级权限\"" w191 {
          tunnel: w192 -> [_ w194]
          frame "一级权限", Default {
          }
          frame "二级权限".."超级权限" {
            n153 = case shown="假" "盐度自动补偿：" {
              tunnel: w194 -> [w198 _]
              frame False {
                n154 = property class="DigNum (严格)"(reference=w198) -> (reference out=w196:refnum<vi>, "Value"=w197:dbl)  [unwired: 1 in, 1 out]
                n155 = call "数字键盘.vi"("OldNumber"=w197) -> ("NewNumber"=w195:dbl)
                n156 = property class="DigNum (严格)"(reference=w196, "Val(Sgnl)"=w195) -> ()  [unwired: 1 in, 2 out]
              }
              frame True {
              }
            }
          }
        }
      }
      event "盐度补偿值": Value Change {
        n157 = event-data() -> ("NewVal"=w199:dbl)  [unwired: 1 in, 5 out]
        n158 = global read "VAR总磷总氮全局变量.vi" "MB session in"() -> (w200:refnum<class "MB_Master.lvclass">)
        n159 = call "盐度补偿值写入.vi"("盐度补偿值"=w199, "MB session in"=w200) -> ()  [unwired: 8 in, 2 out]
      }
      event "跨度值", "零点核查标液浓度", "跨度核查标液浓度", "标样核查标液浓度", "消解时长", "测试流程路径", "盐度自动补偿：", "IP", "PORT", "请选择串口:", "通信方式选择", "简易流程路径", "低量程上限", "零点核查标液偏差", "跨度核查标液偏差", "标样核查标液偏差", "零点核查自动补测", "跨度核查自动补测", "标样核查自动补测": Value Change {
        n160 = event-data() -> ()  [unwired: 1 in, 6 out]
        n161 = global read "VAR总磷总氮全局变量.vi" "权限等级"() -> (w202:enum16{"一级权限", "二级权限", "三级权限", "超级权限"})
        n162 = case shown="\"二级权限\"..\"超级权限\"" w202 {
          tunnel: w203 -> [_ w205]
          tunnel: w201 -> [w204 _]
          frame "一级权限", Default {
            n163 = Set Occurrence(w204) -> ()
          }
          frame "二级权限".."超级权限" {
            n164 = flat-sequence {
              tunnel: w205 -> [w235]
              frame #0 {
                n165 = local read "通信方式选择"() -> (w217:enum16{"串口", "TCP"})
                n166 = property class="Ring (严格)"(reference=w235) -> ("Value"=w234:u16)  [unwired: 1 in, 2 out]
                n167 = local read "盐度自动补偿："() -> (w221:bool)
                n168 = global write "总磷总氮断电保存全局变量.vi" "MB通信方式选择"(w217) -> ()
                n169 = Bundle("水样测试量程模式"="水样测试量程模式", "零点核查量程模式"="零点核查量程模式", "跨度核查量程模式"="跨度核查量程模式", "加标回收量程模式"="加标回收量程模式", "标样核查量程模式"="标样核查量程模式") -> (w223:T14)  [unwired: 1 in]
                n170 = global write "总磷总氮断电保存全局变量.vi" "简易流程路径"("简易流程路径") -> ()
                n171 = global write "总磷总氮断电保存全局变量.vi" "IP"("IP") -> ()
                n172 = global write "总磷总氮断电保存全局变量.vi" "盐度自动补偿："(w221) -> ()
                n173 = global write "总磷总氮断电保存全局变量.vi" "流程路径"("测试流程路径") -> ()
                n174 = global write "总磷总氮断电保存全局变量.vi" "标样核查自动补测"("标样核查自动补测") -> ()
                n175 = global write "总磷总氮断电保存全局变量.vi" "PORT"("PORT") -> ()
                n176 = global write "总磷总氮断电保存全局变量.vi" "跨度核查自动补测"("跨度核查自动补测") -> ()
                n177 = global write "总磷总氮断电保存全局变量.vi" "VISA Resource"("请选择串口:") -> ()
                n178 = global write "总磷总氮断电保存全局变量.vi" "零点核查自动补测"("零点核查自动补测") -> ()
                n179 = To Unsigned Word Integer(number=w223) -> (unsigned 16bit integer=w222:cluster{u16, u16, u16, u16, u16})
                n180 = global read "总磷总氮断电保存全局变量.vi" "低量程上限"() -> (w214:T15)
                n181 = property on="低量程上限" class="DigNum (严格)"() -> ("Value"=w212:dbl)  [unwired: 2 in, 2 out]
                n182 = global read "总磷总氮断电保存全局变量.vi" "质控参数设置"() -> (w229:T16)
                n183 = local read "消解时长"() -> (w216:dbl)
                n184 = case shown="21" w234 {
                  tunnel: "跨度值" -> [_ w249 w263 w276 w289 w302 w315 w328 w341 w355 w369 w382]
                  tunnel: "标样核查标液浓度" -> [_ w246 w260 w273 w286 w299 w312 w325 w338 w352 w366 w379]
                  tunnel: "跨度核查标液浓度" -> [_ w247 w261 w274 w287 w300 w313 w326 w339 w353 w367 w380]
                  tunnel: "零点核查标液浓度" -> [_ w248 w262 w275 w288 w301 w314 w327 w340 w354 w368 w381]
                  tunnel: w229 -> [_ w251 w265 w278 w291 w304 w317 w330 w343 w357 w371 w384]
                  tunnel: w222 -> [_ w245 w259 w272 w285 w298 w311 w324 w337 w350 w364 w378]
                  tunnel: w216 -> [_ w244 w258 _ _ _ _ _ _ w351 w365 _]
                  tunnel: w214 -> [w237 w242 w257 w271 w284 w297 w310 w323 w336 w349 w363 w377]
                  tunnel: [w237 w241 w255 w270 w283 w296 w309 w322 w335 w348 w362 w376] -> w213
                  tunnel: w212 -> [_ w243 w256 w269 w282 w295 w308 w321 w334 w347 w361 w375]
                  tunnel: "标样核查标液偏差" -> [_ w240 w252 w266 w279 w294 w305 w318 w331 w344 w358 w372]
                  tunnel: "跨度核查标液偏差" -> [_ w239 w253 w267 w280 w293 w306 w319 w332 w345 w359 w373]
                  tunnel: "零点核查标液偏差" -> [_ w238 w254 w268 w281 w292 w307 w320 w333 w346 w360 w374]
                  frame 0, Default {
                  }
                  frame 1 {
                    n185 = global write "总磷总氮断电保存全局变量.vi" "总磷自动测试量程配置"(w245) -> ()
                    n186 = global write "总磷总氮断电保存全局变量.vi" "总磷消解时长"(w244) -> ()
                    n187 = Bundle By Name(cluster=w242, "总磷"=w243) -> (w241:T15)
                    n188 = Bundle By Name(cluster=w251, "总磷跨度值"=w249, "总磷零点标准液浓度"=w248, "总磷跨度标准液浓度"=w247, "总磷标准液标准浓度"=w246, "总磷零点标准液偏差"=w238, "总磷跨度标准液偏差"=w239, "总磷标准液标准偏差"=w240) -> (w250:T16)
                    n189 = global write "总磷总氮断电保存全局变量.vi" "质控参数设置"(w250) -> ()
                  }
                  frame 2 {
                    n190 = global write "总磷总氮断电保存全局变量.vi" "总氮自动测试量程配置"(w259) -> ()
                    n191 = global write "总磷总氮断电保存全局变量.vi" "总氮消解时长"(w258) -> ()
                    n192 = Bundle By Name(cluster=w257, "总氮"=w256) -> (w255:T15)
                    n193 = Bundle By Name(cluster=w265, "总氮跨度值"=w263, "总氮零点标准液浓度"=w262, "总氮跨度标准液浓度"=w261, "总氮标准液标准浓度"=w260, "总氮零点标准液偏差"=w254, "总氮跨度标准液偏差"=w253, "总氮标准液标准偏差"=w252) -> (w264:T16)
                    n194 = global write "总磷总氮断电保存全局变量.vi" "质控参数设置"(w264) -> ()
                  }
                  frame 3 {
                    n195 = global write "总磷总氮断电保存全局变量.vi" "氨氮自动测试量程配置"(w272) -> ()
                    n196 = Bundle By Name(cluster=w271, "氨氮"=w269) -> (w270:T15)
                    n197 = Bundle By Name(cluster=w278, "氨氮跨度值"=w276, "氨氮零点标准液浓度"=w275, "氨氮跨度标准液浓度"=w274, "氨氮标准液标准浓度"=w273, "氨氮零点标准液偏差"=w268, "氨氮跨度标准液偏差"=w267, "氨氮标准液标准偏差"=w266) -> (w277:T16)
                    n198 = global write "总磷总氮断电保存全局变量.vi" "质控参数设置"(w277) -> ()
                  }
                  frame 4 {
                    n199 = global write "总磷总氮断电保存全局变量.vi" "磷酸盐自动测试量程配置"(w285) -> ()
                    n200 = Bundle By Name(cluster=w284, "磷酸盐"=w282) -> (w283:T15)
                    n201 = Bundle By Name(cluster=w291, "磷酸盐跨度值"=w289, "磷酸盐零点标准液浓度"=w288, "磷酸盐跨度标准液浓度"=w287, "磷酸盐标准液标准浓度"=w286, "磷酸盐零点标准液偏差"=w281, "磷酸盐跨度标准液偏差"=w280, "磷酸盐标准液标准偏差"=w279) -> (w290:T16)
                    n202 = global write "总磷总氮断电保存全局变量.vi" "质控参数设置"(w290) -> ()
                  }
                  frame 5 {
                    n203 = global write "总磷总氮断电保存全局变量.vi" "硝氮自动测试量程配置"(w298) -> ()
                    n204 = Bundle By Name(cluster=w297, "硝氮"=w295) -> (w296:T15)
                    n205 = Bundle By Name(cluster=w304, "硝氮跨度值"=w302, "硝氮零点标准液浓度"=w301, "硝氮跨度标准液浓度"=w300, "硝氮标准液标准浓度"=w299, "硝氮零点标准液偏差"=w292, "硝氮跨度标准液偏差"=w293, "硝氮标准液标准偏差"=w294) -> (w303:T16)
                    n206 = global write "总磷总氮断电保存全局变量.vi" "质控参数设置"(w303) -> ()
                  }
                  frame 6 {
                    n207 = global write "总磷总氮断电保存全局变量.vi" "亚硝氮自动测试量程配置"(w311) -> ()
                    n208 = Bundle By Name(cluster=w310, "亚硝氮"=w308) -> (w309:T15)
                    n209 = Bundle By Name(cluster=w317, "亚硝氮跨度值"=w315, "亚硝氮零点标准液浓度"=w314, "亚硝氮跨度标准液浓度"=w313, "亚硝氮标准液标准浓度"=w312, "亚硝氮零点标准液偏差"=w307, "亚硝氮跨度标准液偏差"=w306, "亚硝氮标准液标准偏差"=w305) -> (w316:T16)
                    n210 = global write "总磷总氮断电保存全局变量.vi" "质控参数设置"(w316) -> ()
                  }
                  frame 7 {
                    n211 = global write "总磷总氮断电保存全局变量.vi" "硅酸盐自动测试量程配置"(w324) -> ()
                    n212 = Bundle By Name(cluster=w323, "硅酸盐"=w321) -> (w322:T15)
                    n213 = Bundle By Name(cluster=w330, "硅酸盐跨度值"=w328, "硅酸盐零点标准液浓度"=w327, "硅酸盐跨度标准液浓度"=w326, "硅酸盐标准液标准浓度"=w325, "硅酸盐零点标准液偏差"=w320, "硅酸盐跨度标准液偏差"=w319, "硅酸盐标准液标准偏差"=w318) -> (w329:T16)
                    n214 = global write "总磷总氮断电保存全局变量.vi" "质控参数设置"(w329) -> ()
                  }
                  frame 8 {
                    n215 = global write "总磷总氮断电保存全局变量.vi" "硫化物自动测试量程配置"(w337) -> ()
                    n216 = Bundle By Name(cluster=w336, "硫化物"=w334) -> (w335:T15)
                    n217 = Bundle By Name(cluster=w343, "硫化物跨度值"=w341, "硫化物零点标准液浓度"=w340, "硫化物跨度标准液浓度"=w339, "硫化物标准液标准浓度"=w338, "硫化物零点标准液偏差"=w333, "硫化物跨度标准液偏差"=w332, "硫化物标准液标准偏差"=w331) -> (w342:T16)
                    n218 = global write "总磷总氮断电保存全局变量.vi" "质控参数设置"(w342) -> ()
                  }
                  frame 22 {
                    n219 = global write "总磷总氮断电保存全局变量.vi" "COD自动测试量程配置"(w350) -> ()
                    n220 = global write "总磷总氮断电保存全局变量.vi" "CODcr消解时长"(w351) -> ()
                    n221 = Bundle By Name(cluster=w349, "COD"=w347) -> (w348:T15)
                    n222 = Bundle By Name(cluster=w357, "COD跨度值"=w355, "COD零点标准液浓度"=w354, "COD跨度标准液浓度"=w353, "COD标准液标准浓度"=w352, "COD零点标准液偏差"=w346, "COD跨度标准液偏差"=w345, "COD标准液标准偏差"=w344) -> (w356:T16)
                    n223 = global write "总磷总氮断电保存全局变量.vi" "质控参数设置"(w356) -> ()
                  }
                  frame 21 {
                    n224 = global write "总磷总氮断电保存全局变量.vi" "CODMn自动测试量程配置"(w364) -> ()
                    n225 = global write "总磷总氮断电保存全局变量.vi" "CODmn消解时长"(w365) -> ()
                    n226 = Bundle By Name(cluster=w363, "CODMn"=w361) -> (w362:T15)
                    n227 = Bundle By Name(cluster=w371, "CODMn跨度值"=w369, "CODMn零点标准液浓度"=w368, "CODMn跨度标准液浓度"=w367, "CODMn标准液标准浓度"=w366, "CODMn零点标准液偏差"=w360, "CODMn跨度标准液偏差"=w359, "CODMn标准液标准偏差"=w358) -> (w370:T16)
                    n228 = global write "总磷总氮断电保存全局变量.vi" "质控参数设置"(w370) -> ()
                  }
                  frame 50 {
                    n229 = global write "总磷总氮断电保存全局变量.vi" "氟化物自动测试量程配置"(w378) -> ()
                    n230 = Bundle By Name(cluster=w377, "氟化物"=w375) -> (w376:T15)
                    n231 = Bundle By Name(cluster=w384, "氟化物跨度值"=w382, "氟化物零点标准液浓度"=w381, "氟化物跨度标准液浓度"=w380, "氟化物标准液标准浓度"=w379, "氟化物零点标准液偏差"=w374, "氟化物跨度标准液偏差"=w373, "氟化物标准液标准偏差"=w372) -> (w383:T16)
                    n232 = global write "总磷总氮断电保存全局变量.vi" "质控参数设置"(w383) -> ()
                  }
                }
                n233 = global write "总磷总氮断电保存全局变量.vi" "低量程上限"(w213) -> ()
              }
              frame #1 {
                n234 = Get Date/Time In Seconds() -> (seconds since 1Jan1904=w387:timestamp)
                n235 = property on="参数下拉列表" class="Ring (严格)"() -> ("RingText.Text"=w385:string)  [unwired: 2 in, 2 out]
                n236 = Bundle By Name(cluster=T8 {"时间"=timestamp(0 s since 1904-01-01), "参数"="", "日志信息"="", "流程参数"=""} ("data in"), "时间"=w387, "参数"=w385, "日志信息"="参数变更") -> (w388:T8)
                n237 = call "总磷总氮操作日志.vi"("data in"=w388) -> ()  [unwired: 10 in, 1 out]
                n238 = call "仪器配置写入.vi"() -> ()  [unwired: 11 in, 1 out]
              }
            }
          }
        }
      }
      event "通讯连接": Value Change {
        n239 = event-data() -> ("NewVal"=w390:bool)  [unwired: 1 in, 5 out]
        n240 = Flush Queue(queue=w391) -> (queue out=w392:refnum<queue>)  [unwired: 1 in, 2 out]
        n241 = case shown="假" w390 {
          tunnel: w392 -> [w393 w395]
          frame False {
            n242 = Enqueue Element At Opposite End(queue=w393, element=cluster{"命令":string, "data":variant} {"命令"="停用模块", "data"=variant} ("元素")) -> ()  [unwired: 2 in, 3 out]
          }
          frame True {
            n243 = Enqueue Element At Opposite End(queue=w395, element=cluster{"命令":string, "data":variant} {"命令"="启用模块", "data"=variant} ("元素")) -> ()  [unwired: 2 in, 3 out]
          }
        }
      }
    }
  }
  n244 = while {
    tunnel: w7 -> [w407]
    tunnel: w8 -> [w406]
    tunnel: w9 -> [w405]
    tunnel: w6 -> [w404]
    stop <- FALSE stop-if-true
    n245 = Wait on Occurrence(2:w404) -> (0:w398:bool)  [unwired: 2 in]
    n246 = flat-sequence {
      tunnel: w407 -> [w414]
      tunnel: w406 -> [w413]
      tunnel: w405 -> [w412]
      tunnel: [w411] -> w401
      tunnel: [w410] -> w400
      tunnel: [w409] -> w399
      tunnel: w398 -> [_]
      frame #0 {
        n247 = property class="Enum (严格)"(reference=w413) -> ("Value"=w410:enum16{"低量程", "高量程"})  [unwired: 1 in, 2 out]
        n248 = property class="Ring (严格)"(reference=w414) -> ("Value"=w411:u16)  [unwired: 1 in, 2 out]
        n249 = property class="Enum (严格)"(reference=w412) -> ("Value"=w409:T1)  [unwired: 1 in, 2 out]
      }
    }
    n250 = flat-sequence {
      tunnel: [w417] -> w403
      tunnel: [w416] -> w402
      tunnel: w401 -> [w415]
      tunnel: w400 -> [w417]
      tunnel: w399 -> [w416]
      tunnel: [w415] -> w397
      tunnel: w403 -> [w436]
      tunnel: w402 -> [w437]
      tunnel: w397 -> [w435]
      frame #0 {
      }
      frame #1 {
        n251 = call "量程参数读取.vi"("测量参数"=w435) -> ("error out"=w426:errorcluster, "量程参数读取"=w434:T7)  [unwired: 9 in]
        n252 = Unbundle By Name(w434) -> ("测量精度"=→"测量精度":u16, "检出限"=→"检出限":dbl, "上限"=→"高量程上限":dbl, "下限"=→"量程下限":dbl, "阈值（低->高）"=→"阈值（低->高）":dbl, "阈值（高->低）"=→"阈值（高->低）":dbl, "稀释度"=→"稀释度":dbl)
        n253 = call "公式读取.vi"("error in (no error)"=w426, "量程"=w436, "测量模式"=w437, "测量参数"=w435) -> ("error out"=w420:errorcluster, "公式"=w425:cluster{"X^2":dbl, "X":dbl, "b":dbl})  [unwired: 6 in]
        n254 = Unbundle By Name(w425) -> ("X^2"=→"二次多项式系数":dbl, "X"=→"曲线斜率":dbl, "b"=→"曲线截距":dbl)
        n255 = global read "VAR总磷总氮全局变量.vi" "MB session in"() -> (w419:refnum<class "MB_Master.lvclass">)
        n256 = case shown="1, 2, 21, 22" w435 {
          tunnel: [_ w440] -> w421
          tunnel: [w438 w446] -> _
          tunnel: w420 -> [w438 w441]
          tunnel: w419 -> [_ w444]
          tunnel: [_ w445] -> w418
          frame 0, Default {
          }
          frame 1, 2, 21, 22 {
            n257 = call "版本判断.vi"() -> ("仪器版本"=w443:T9)  [unwired: 11 in]
            n258 = case shown="\"V4.2版\"" w443 {
              tunnel: [w452 w456 w461 w467] -> w442
              tunnel: w444 -> [w451 w457 w462 w468]
              tunnel: [w448 w454 w459 w465] -> w440
              tunnel: w441 -> [w450 _ _ w464]
              tunnel: [w447 w453 w458 w463] -> w439
              frame "V3.1版", Default {
                n259 = call "读取V3.1外设配置.vi"("error in (no error)"=w450, "MB session in"=w451) -> ("error out"=w452:errorcluster, "外设配置"=w449:T10, "MB session out"=w447:refnum<class "MB_Master.lvclass">)  [unwired: 7 in]
                n260 = Unbundle By Name(w449) -> ("消解温度下限"=w448:sgl)
              }
              frame "V4版" {
                n261 = call "读取V4版外设配置.vi"("MB session in"=w457) -> ("error out"=w456:errorcluster, "外设配置"=w455:T11, "MB session out"=w453:refnum<class "MB_Master.lvclass">)  [unwired: 8 in]
                n262 = Unbundle By Name(w455) -> ("消解温度下限"=w454:sgl)
              }
              frame "V4.2版" {
                n263 = call "读取V4.2版外设配置.vi"("MB session in"=w462) -> ("error out"=w461:errorcluster, "外设配置"=w460:T12, "MB session out"=w458:refnum<class "MB_Master.lvclass">)  [unwired: 8 in]
                n264 = Unbundle By Name(w460) -> ("消解温度"=w459:sgl)
              }
              frame "V3版" {
                n265 = call "读取V3外设配置.vi"("error in (no error)"=w464, "MB session in"=w468) -> ("error out"=w467:errorcluster, "外设配置"=w466:T13, "MB session out"=w463:refnum<class "MB_Master.lvclass">)  [unwired: 7 in]
                n266 = Unbundle By Name(w466) -> ("消解温度下限"=w465:sgl)
              }
            }
            n267 = call "盐度补偿值读取.vi"("Error in"=w442, "MB session in"=w439) -> ("error out"=w446:errorcluster, "盐度补偿值"=w445:sgl)  [unwired: 7 in, 1 out]
          }
        }
        "消解温度" <- w421
        "盐度补偿值" <- w418
      }
      frame #2 {
        n268 = Format Date/Time String() -> (date/time string=→"数据刷新时间":string)  [unwired: 3 in]
      }
    }
  }
  n269 = while {
    tunnel: w7 -> [w480]
    stop <- FALSE stop-if-true
    n270 = global read "总磷总氮断电保存全局变量.vi" "盐度自动补偿："() -> (w495:bool)
    n271 = property class="Ring (严格)"(reference=w480) -> ("Value"=w479:u16)  [unwired: 1 in, 2 out]
    n272 = global read "总磷总氮断电保存全局变量.vi" "跨度核查自动补测"() -> (w470:bool)
    n273 = global read "总磷总氮断电保存全局变量.vi" "MB通信方式选择"() -> (w494:enum16{"串口", "TCP"})
    n274 = global read "总磷总氮断电保存全局变量.vi" "VISA Resource"() -> (w499:refnum<visa-resource-name>)
    n275 = global read "总磷总氮断电保存全局变量.vi" "简易流程路径"() -> (w478:path)
    n276 = global read "总磷总氮断电保存全局变量.vi" "零点核查自动补测"() -> (w472:bool)
    n277 = global read "总磷总氮断电保存全局变量.vi" "标样核查自动补测"() -> (w471:bool)
    n278 = global read "总磷总氮断电保存全局变量.vi" "流程路径"() -> (w496:path)
    n279 = global read "总磷总氮断电保存全局变量.vi" "PORT"() -> (w498:string)
    n280 = local write "盐度自动补偿："(w495) -> ()
    n281 = global read "总磷总氮断电保存全局变量.vi" "质控参数设置"() -> (w489:T16)
    n282 = global read "总磷总氮断电保存全局变量.vi" "低量程上限"() -> (w477:T15)
    n283 = local write "跨度核查自动补测"(w470) -> ()
    n284 = local write "通信方式选择"(w494) -> ()
    n285 = local write "请选择串口:"(w499) -> ()
    n286 = local write "简易流程路径"(w478) -> ()
    n287 = local write "零点核查自动补测"(w472) -> ()
    n288 = local write "标样核查自动补测"(w471) -> ()
    n289 = local write "测试流程路径"(w496) -> ()
    n290 = local write "PORT"(w498) -> ()
    n291 = case shown="21" w479 {
      tunnel: [_ w514 w526 w537 w548 w559 w570 w581 w592 w604 w615 w627] -> w487
      tunnel: [_ w513 w525 _ _ _ _ _ _ w603 _ w616] -> w488
      tunnel: w489 -> [_ w512 w524 w536 w547 w558 w569 w580 w591 w602 w614 w626]
      tunnel: [_ w511 w523 w535 w546 w557 w568 w579 w590 w601 w613 w625] -> w490
      tunnel: [_ w510 w522 w534 w545 w556 w567 w578 w589 w600 w612 w624] -> w491
      tunnel: [_ w509 w521 w533 w544 w555 w566 w577 w588 w599 w611 w623] -> w492
      tunnel: [_ w508 w520 w532 w543 w554 w565 w576 w587 w598 w610 w622] -> w493
      tunnel: w477 -> [_ w507 w519 w531 w542 w553 w564 w575 w586 w597 w609 w621]
      tunnel: [0.0 ("COD") w506 w518 w530 w541 w552 w563 w574 w585 w596 w608 w620] -> w476
      tunnel: [_ w505 w517 w529 w540 w551 w562 w573 w584 w595 w607 w619] -> w475
      tunnel: [_ w504 w516 w528 w539 w550 w561 w572 w583 w594 w606 w618] -> w474
      tunnel: [_ w503 w515 w527 w538 w549 w560 w571 w582 w593 w605 w617] -> w473
      frame Default {
      }
      frame 1 {
        n292 = Unbundle By Name(w512) -> ("总磷跨度值"=w511:dbl, "总磷零点标准液浓度"=w510:dbl, "总磷跨度标准液浓度"=w509:dbl, "总磷标准液标准浓度"=w508:dbl, "总磷零点标准液偏差"=w505:dbl, "总磷跨度标准液偏差"=w504:dbl, "总磷标准液标准偏差"=w503:dbl)
        n293 = Unbundle By Name(w507) -> ("总磷"=w506:dbl)
        n294 = global read "总磷总氮断电保存全局变量.vi" "总磷消解时长"() -> (w513:dbl)
        n295 = global read "总磷总氮断电保存全局变量.vi" "总磷自动测试量程配置"() -> (w514:T17)
      }
      frame 2 {
        n296 = Unbundle By Name(w524) -> ("总氮跨度值"=w523:dbl, "总氮零点标准液浓度"=w522:dbl, "总氮跨度标准液浓度"=w521:dbl, "总氮标准液标准浓度"=w520:dbl, "总氮零点标准液偏差"=w517:dbl, "总氮跨度标准液偏差"=w516:dbl, "总氮标准液标准偏差"=w515:dbl)
        n297 = Unbundle By Name(w519) -> ("总氮"=w518:dbl)
        n298 = global read "总磷总氮断电保存全局变量.vi" "总氮消解时长"() -> (w525:dbl)
        n299 = global read "总磷总氮断电保存全局变量.vi" "总氮自动测试量程配置"() -> (w526:T17)
      }
      frame 3 {
        n300 = Unbundle By Name(w536) -> ("氨氮跨度值"=w535:dbl, "氨氮零点标准液浓度"=w534:dbl, "氨氮跨度标准液浓度"=w533:dbl, "氨氮标准液标准浓度"=w532:dbl, "氨氮零点标准液偏差"=w529:dbl, "氨氮跨度标准液偏差"=w528:dbl, "氨氮标准液标准偏差"=w527:dbl)
        n301 = Unbundle By Name(w531) -> ("氨氮"=w530:dbl)
        n302 = global read "总磷总氮断电保存全局变量.vi" "氨氮自动测试量程配置"() -> (w537:T17)
      }
      frame 4 {
        n303 = Unbundle By Name(w547) -> ("磷酸盐跨度值"=w546:dbl, "磷酸盐零点标准液浓度"=w545:dbl, "磷酸盐跨度标准液浓度"=w544:dbl, "磷酸盐标准液标准浓度"=w543:dbl, "磷酸盐零点标准液偏差"=w540:dbl, "磷酸盐跨度标准液偏差"=w539:dbl, "磷酸盐标准液标准偏差"=w538:dbl)
        n304 = Unbundle By Name(w542) -> ("磷酸盐"=w541:dbl)
        n305 = global read "总磷总氮断电保存全局变量.vi" "磷酸盐自动测试量程配置"() -> (w548:T17)
      }
      frame 5 {
        n306 = Unbundle By Name(w558) -> ("硝氮跨度值"=w557:dbl, "硝氮零点标准液浓度"=w556:dbl, "硝氮跨度标准液浓度"=w555:dbl, "硝氮标准液标准浓度"=w554:dbl, "硝氮零点标准液偏差"=w551:dbl, "硝氮跨度标准液偏差"=w550:dbl, "硝氮标准液标准偏差"=w549:dbl)
        n307 = Unbundle By Name(w553) -> ("硝氮"=w552:dbl)
        n308 = global read "总磷总氮断电保存全局变量.vi" "硝氮自动测试量程配置"() -> (w559:T17)
      }
      frame 6 {
        n309 = Unbundle By Name(w569) -> ("亚硝氮跨度值"=w568:dbl, "亚硝氮零点标准液浓度"=w567:dbl, "亚硝氮跨度标准液浓度"=w566:dbl, "亚硝氮标准液标准浓度"=w565:dbl, "亚硝氮零点标准液偏差"=w562:dbl, "亚硝氮跨度标准液偏差"=w561:dbl, "亚硝氮标准液标准偏差"=w560:dbl)
        n310 = Unbundle By Name(w564) -> ("亚硝氮"=w563:dbl)
        n311 = global read "总磷总氮断电保存全局变量.vi" "亚硝氮自动测试量程配置"() -> (w570:T17)
      }
      frame 7 {
        n312 = Unbundle By Name(w580) -> ("硅酸盐跨度值"=w579:dbl, "硅酸盐零点标准液浓度"=w578:dbl, "硅酸盐跨度标准液浓度"=w577:dbl, "硅酸盐标准液标准浓度"=w576:dbl, "硅酸盐零点标准液偏差"=w573:dbl, "硅酸盐跨度标准液偏差"=w572:dbl, "硅酸盐标准液标准偏差"=w571:dbl)
        n313 = Unbundle By Name(w575) -> ("硅酸盐"=w574:dbl)
        n314 = global read "总磷总氮断电保存全局变量.vi" "硅酸盐自动测试量程配置"() -> (w581:T17)
      }
      frame 8 {
        n315 = Unbundle By Name(w591) -> ("硫化物跨度值"=w590:dbl, "硫化物零点标准液浓度"=w589:dbl, "硫化物跨度标准液浓度"=w588:dbl, "硫化物标准液标准浓度"=w587:dbl, "硫化物零点标准液偏差"=w584:dbl, "硫化物跨度标准液偏差"=w583:dbl, "硫化物标准液标准偏差"=w582:dbl)
        n316 = Unbundle By Name(w586) -> ("硫化物"=w585:dbl)
        n317 = global read "总磷总氮断电保存全局变量.vi" "硫化物自动测试量程配置"() -> (w592:T17)
      }
      frame 22 {
        n318 = Unbundle By Name(w602) -> ("COD跨度值"=w601:dbl, "COD零点标准液浓度"=w600:dbl, "COD跨度标准液浓度"=w599:dbl, "COD标准液标准浓度"=w598:dbl, "COD零点标准液偏差"=w595:dbl, "COD跨度标准液偏差"=w594:dbl, "COD标准液标准偏差"=w593:dbl)
        n319 = Unbundle By Name(w597) -> ("COD"=w596:dbl)
        n320 = global read "总磷总氮断电保存全局变量.vi" "CODcr消解时长"() -> (w603:dbl)
        n321 = global read "总磷总氮断电保存全局变量.vi" "COD自动测试量程配置"() -> (w604:T17)
      }
      frame 50 {
        n322 = Unbundle By Name(w614) -> ("氟化物跨度值"=w613:dbl, "氟化物零点标准液浓度"=w612:dbl, "氟化物跨度标准液浓度"=w611:dbl, "氟化物标准液标准浓度"=w610:dbl, "氟化物零点标准液偏差"=w607:dbl, "氟化物跨度标准液偏差"=w606:dbl, "氟化物标准液标准偏差"=w605:dbl)
        n323 = Unbundle By Name(w609) -> ("氟化物"=w608:dbl)
        n324 = global read "总磷总氮断电保存全局变量.vi" "氟化物自动测试量程配置"() -> (w615:T17)
      }
      frame 21 {
        n325 = Unbundle By Name(w626) -> ("CODMn跨度值"=w625:dbl, "CODMn零点标准液浓度"=w624:dbl, "CODMn跨度标准液浓度"=w623:dbl, "CODMn标准液标准浓度"=w622:dbl, "CODMn零点标准液偏差"=w619:dbl, "CODMn跨度标准液偏差"=w618:dbl, "CODMn标准液标准偏差"=w617:dbl)
        n326 = Unbundle By Name(w621) -> ("CODMn"=w620:dbl)
        n327 = global read "总磷总氮断电保存全局变量.vi" "CODMn自动测试量程配置"() -> (w627:T17)
        n328 = global read "总磷总氮断电保存全局变量.vi" "CODcr消解时长"() -> (w616:dbl)
      }
    }
    "消解时长" <- w488
    "低量程上限" <- w476
    n329 = global read "总磷总氮断电保存全局变量.vi" "IP"() -> (w497:string)
    n330 = local write "IP"(w497) -> ()
    n331 = Wait (ms)(milliseconds to wait=u32 1000 ("等待时间（毫秒）")) -> ()  [unwired: 1 out]
    n332 = local write "跨度值"(w490) -> ()
    n333 = local write "零点核查标液浓度"(w491) -> ()
    n334 = local write "跨度核查标液浓度"(w492) -> ()
    n335 = local write "标样核查标液浓度"(w493) -> ()
    n336 = local write "零点核查标液偏差"(w475) -> ()
    n337 = local write "跨度核查标液偏差"(w474) -> ()
    n338 = local write "标样核查标液偏差"(w473) -> ()
    n339 = To Unsigned Word Integer(number=w487) -> (unsigned 16bit integer=w486:T18)
    n340 = Unbundle By Name(w486) -> ("水样测试量程模式"=w485:u16, "空白核查量程模式"=w483:u16, "跨度核查量程模式"=w482:u16, "加标回收量程模式"=w481:u16, "标样核查量程模式"=w484:u16)
    n341 = local write "水样测试量程模式"(w485) -> ()
    n342 = local write "零点核查量程模式"(w483) -> ()
    n343 = local write "跨度核查量程模式"(w482) -> ()
    n344 = local write "加标回收量程模式"(w481) -> ()
    n345 = local write "标样核查量程模式"(w484) -> ()
  }
